vi "Run.vi"(4 "Dispense?":bool, 6 "Pickup_Test_Number":dbl, 7 "Database Entry in":refnum<class "Database Entry.lvclass">, 8 "error in (no error)":errorcluster, 9 "Assembly Type":string, 10 "Control In":T1={"I-O.lvclass"=refnum, "Gantry"=refnum, "Dispenser"="COM1"}, 11 "Assembly In":refnum<class "Assembly Run.lvclass">) -> (0 "error out":errorcluster, 2 "Control Out":T1={"I-O.lvclass"=refnum, "Gantry"=refnum, "Dispenser"="COM1"}, 3 "Assembly Out":refnum<class "Assembly Run.lvclass">, 5 "Database Entry out":refnum<class "Database Entry.lvclass">)   [LabVIEW 2021, in "Assembly Run.lvclass"]
uses:
  Assembly Run.lvclass
  Controller/Controllers.ctl
  Controller/I-O/I-O.lvclass
  C:/Program Files (x86)/Aerotech/A3200/LabVIEW/2010/Bin/Aerotech.A3200.dll
  Program Files (x86)/Aerotech/A3200/LabVIEW/2010/Bin/Aerotech.A3200.dll
  Database Entry/Database Entry.lvclass
  Assembly Run.lvclass/Assembly Run.ctl
  Workspace/Fixture.lvclass
  Routine/Routine.lvclass
  Controller/Motion/Motion.lvclass
  Controller/Motion/A3200/A3200.lvclass
  Drivers/Aerotech A3200/Aerotech.lvlib
  Controller/Controller.lvclass
panel:
  out "Program End?":bool
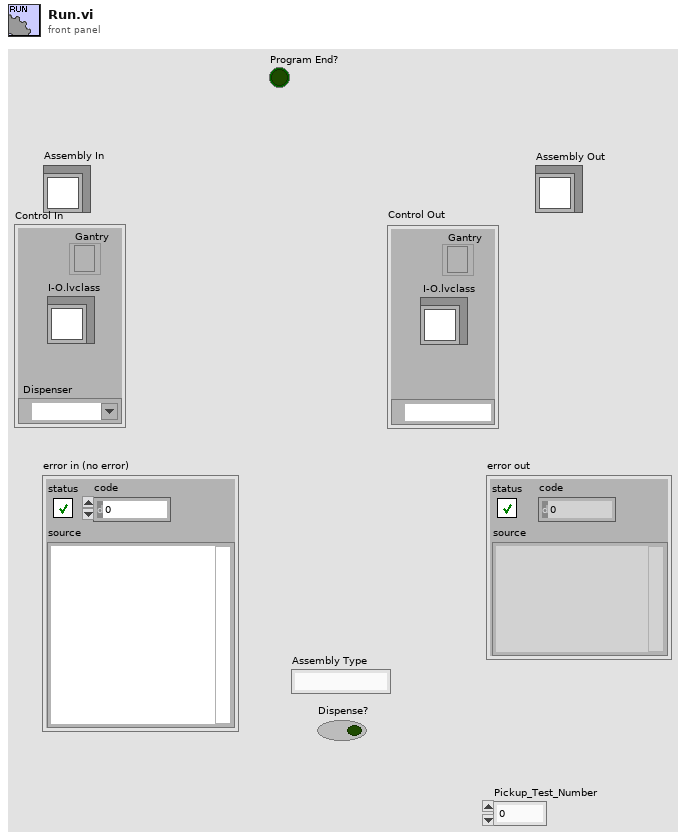
[diagram p1: front panel]
types:
  T1 = typedef "Controller.lvclass/Controllers.ctl" = cluster{"I-O.lvclass":refnum<class "I-O.lvclass">, "Gantry":refnum<k24>, "Dispenser":refnum<visa-resource-name>}
  T2 = typedef "Fixture.lvclass/Workspace.ctl" = cluster{"XYZTheta":dbl[], "Workspace Valve":i32, "Workspace Sensor":i32, "Tray Number":i32, "Position":i32, "Assembly Type":string, "Numeric":dbl, "First Pos":i32}
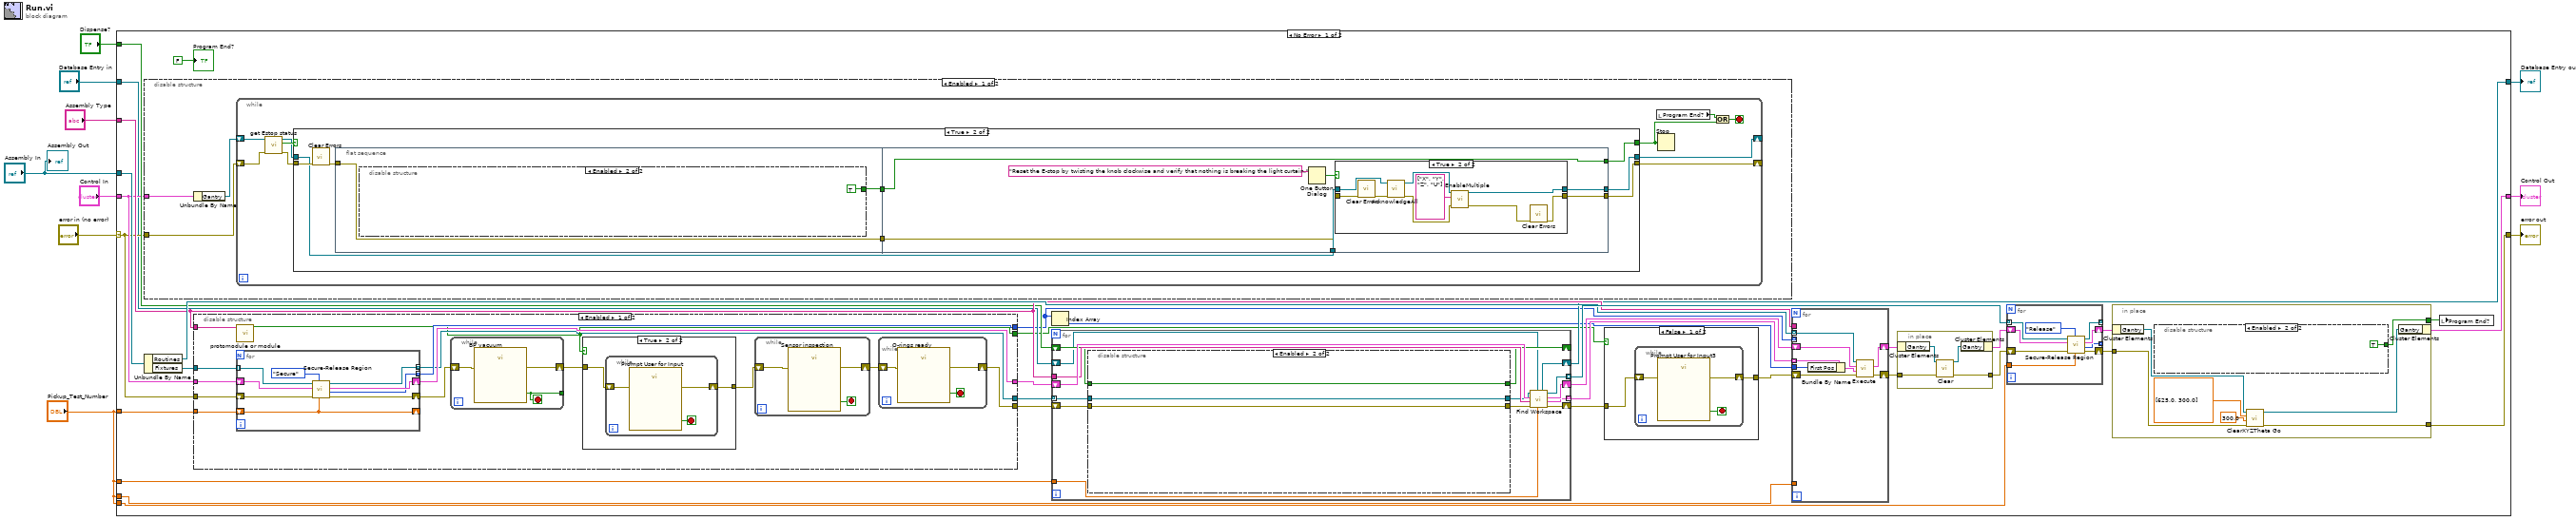
[diagram p0: block diagram]
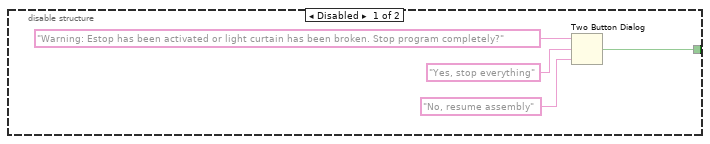
[diagram p4: hidden frame]
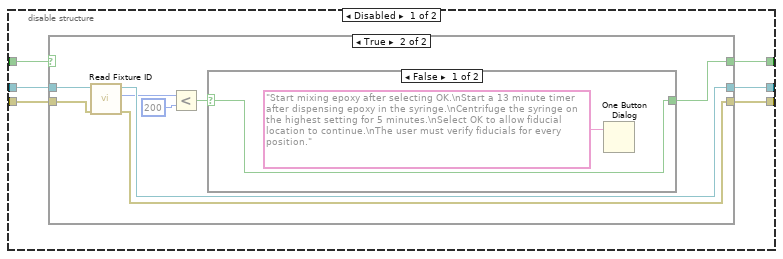
[diagram p7: hidden frame]
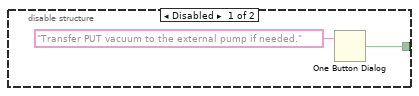
[diagram p10: hidden frame]
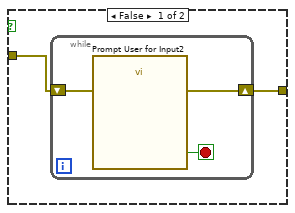
[diagram p11: hidden frame]
diagram:
  n1 = case shown="No Error" "error in (no error)" {
    selector: "error in (no error)" -> [w20 w215]
    tunnel: [w25 w215] -> w9
    tunnel: [w30 w214] -> w8
    tunnel: "Assembly In" -> [w40 _]
    tunnel: "Control In" -> [w21 w214]
    tunnel: "Assembly Type" -> [w23 _]
    tunnel: "Pickup_Test_Number" -> [w36 _]
    tunnel: "Pickup_Test_Number" -> [w34 _]
    tunnel: "Pickup_Test_Number" -> [w35 _]
    tunnel: "Pickup_Test_Number" -> [w33 _]
    tunnel: "Dispense?" -> [w22 _]
    tunnel: "Database Entry in" -> [w17 w213]
    tunnel: [w16 w213] -> w1
    frame No Error {
      n2 = disable-structure shown="Enabled" {
        disable-tunnel: w21 -> [w53 _]
        disable-tunnel: w20 -> [w51 _]
        frame Enabled {
          n3 = Unbundle By Name(w53) -> ("Gantry"=w52:refnum<k24>)
          n4 = while {
            shift-right: [w57] -> _
            shift-left: w52 -> [w63]
            shift-right: [w59] -> _
            shift-left: w51 -> [w62]
            stop <- w56 stop-if-true
            n5 = call "get Estop status.vi"("error in (no error)"=w62, "controller in"=w63) -> ("error out"=w60:errorcluster, "Estop?"=w61:bool, "controller out"=w58:refnum<k24>)  [unwired: 7 in]
            n6 = case shown="True" w61 {
              selector: w61 -> [w65 _]
              tunnel: w60 -> [w66 w74]
              tunnel: [w66 w67] -> w59
              tunnel: [w65 w73] -> w55
              tunnel: w58 -> [w64 w69]
              tunnel: [w64 w68] -> w57
              frame False {
              }
              frame True {
                n7 = call <vilib>:"Clear Errors.vi"("error in (no error)"=w74) -> ("error out"=w71:errorcluster)  [unwired: 5 in, 1 out]
                n8 = flat-sequence {
                  tunnel: [w76] -> w72
                  tunnel: w71 -> [w75]
                  tunnel: [w75] -> w70
                  tunnel: [w88] -> w73
                  tunnel: w72 -> [w88]
                  tunnel: w70 -> [w82]
                  tunnel: w69 -> [w85]
                  tunnel: [w84] -> w68
                  tunnel: [w83] -> w67
                  frame #0 {
                    n9 = disable-structure shown="Enabled" {
                      disable-tunnel: [w77 TRUE ("T button?")] -> w76
                      frame Disabled {
                        n10 = Two Button Dialog(message="Warning: Estop has been activated or light curtain has been broken. Stop program completely?", 1:"No, resume assembly" ("F button name (\"Cancel\")"), 2:"Yes, stop everything" ("T button name (\"OK\")")) -> (T button?=w77:bool)
                      }
                      frame Enabled {
                      }
                    }
                  }
                  frame #1 {
                    n11 = One Button Dialog(message="Reset the E-stop by twisting the knob clockwise and verify that nothing is breaking the light curtain.") -> (true=w86:bool)  [unwired: 1 in]
                    n12 = case shown="True" w86 {
                      tunnel: w85 -> [w90 w98]
                      tunnel: w82 -> [w89 w97]
                      tunnel: [w90 w94] -> w84
                      tunnel: [w89 w91] -> w83
                      frame False {
                      }
                      frame True {
                        n13 = call <vilib>:"Clear Errors.vi"("error in (no error)"=w97) -> ("error out"=w99:errorcluster)  [unwired: 5 in, 1 out]
                        n14 = call "AcknowledgeAll.vi"("error in (no error)"=w99, "controller in"=w98) -> ("error out"=w95:errorcluster, "controller out"=w96:refnum<k24>)  [unwired: 8 in]
                        n15 = call "EnableMultiple.vi"("error in (no error)"=w95, "axis names"=string[] ["X", "Y", "Z", "U"], "controller in"=w96) -> ("error out"=w92:errorcluster, "controller out"=w94:refnum<k24>)  [unwired: 7 in]
                        n16 = call <vilib>:"Clear Errors.vi"("error in (no error)"=w92) -> ("error out"=w91:errorcluster)  [unwired: 5 in, 1 out]
                      }
                    }
                  }
                }
              }
            }
            n17 = local read "Program End?"() -> (w54:bool)
            n18 = Stop(stop? (T)=w55) -> ()
            n19 = Or(x=w54, y=w55) -> (x .or. y?=w56:bool)
          }
        }
        frame Disabled {
        }
      }
      n20 = Unbundle By Name(w40) -> ("Routines"=w24:refnum<class "Routine.lvclass">[], "Fixtures"=w41:refnum<class "Fixture.lvclass">[])
      n21 = disable-structure shown="Enabled" {
        disable-tunnel: [w152 w191] -> w43
        disable-tunnel: w41 -> [w161 w191]
        disable-tunnel: w21 -> [w160 w190]
        disable-tunnel: [w159 w190] -> w37
        disable-tunnel: [w158 _] -> w12
        disable-tunnel: w34 -> [w157 _]
        disable-tunnel: w20 -> [w156 _]
        disable-tunnel: [w149 _] -> w29
        disable-tunnel: w23 -> [w151 _]
        disable-tunnel: [w148 _] -> w13
        frame Enabled {
          n22 = for {
            tunnel: [w189] -> w152 mode=indexing
            tunnel: w161 -> [w188] mode=indexing
            shift-right: [w186] -> w159
            shift-left: w160 -> [w187]
            tunnel: [w184] -> w158 mode=indexing
            shift-right: [w183] -> _
            shift-left: w157 -> [w183]
            shift-right: [w182] -> w155
            shift-left: w156 -> [w181]
            n23 = call-dynamic "Secure-Release Region.vi"("Test Run Number"=w183, "Action"=enum16{"Secure", "Release"}."Secure", "error in (no error)"=w181, "Control In"=w187, "Fixture in"=w188) -> ("error out"=w182:errorcluster, "Position"=w184:i32, "Control Out"=w186:T1, "Fixture out"=w189:refnum<class "Fixture.lvclass">)  [unwired: 3 in]
          }
          n24 = call "protomodule or module.vi"("assembly type"=w151) -> ("protomodule? (T)"=w148:bool)  [unwired: 10 in]
          n25 = while {
            tunnel: [w180] -> _
            shift-right: [w178] -> w154
            shift-left: w155 -> [w179]
            stop <- w180 stop-if-true
            n26 = call "BP vacuum"("error in (no error)"=w179) -> ("BP vacuum is on?"=w180:bool, "error out"=w178:errorcluster)  [unwired: 16 in, 1 out]
          }
          n27 = case shown="True" w148 {
            tunnel: w154 -> [w169 w174]
            tunnel: [w168 w173] -> w153
            frame False {
              n28 = while {
                shift-right: [w171] -> w168
                shift-left: w169 -> [w172]
                stop <- w170 stop-if-true
                n29 = call "Prompt User for Input2"("error in (no error)"=w172) -> ("HB backlighting on?"=w170:bool, "error out"=w171:errorcluster)  [unwired: 16 in, 1 out]
              }
            }
            frame True {
              n30 = while {
                shift-right: [w175] -> w173
                shift-left: w174 -> [w176]
                stop <- w177 stop-if-true
                n31 = call "Prompt User for Input"("error in (no error)"=w176) -> ("BP paper is removed?"=w177:bool, "error out"=w175:errorcluster)  [unwired: 16 in, 1 out]
              }
            }
          }
          n32 = while {
            shift-right: [w163] -> w150
            shift-left: w153 -> [w162]
            stop <- w164 stop-if-true
            n33 = call "Sensor inspection"("error in (no error)"=w162) -> ("Sensors inspected?"=w164:bool, "error out"=w163:errorcluster)  [unwired: 16 in, 1 out]
          }
          n34 = while {
            shift-right: [w166] -> w149
            shift-left: w150 -> [w165]
            stop <- w167 stop-if-true
            n35 = call "O-rings ready"("error in (no error)"=w165) -> ("O-rings ready?"=w167:bool, "error out"=w166:errorcluster)  [unwired: 16 in, 1 out]
          }
        }
        frame Disabled {
        }
      }
      n36 = Index Array(array=w12) -> (element=w11:i32)  [unwired: 1 in]
      n37 = for {
        tunnel: w43 -> [w107] mode=indexing
        tunnel: [w110] -> w44 mode=indexing
        tunnel: [w114] -> w32 mode=indexing
        shift-right: [w112] -> w39
        shift-left: w37 -> [w113]
        tunnel: w23 -> [w111]
        tunnel: w33 -> [w109]
        shift-right: [w108] -> w15
        shift-left: w29 -> [w105]
        shift-right: [w102] -> _
        shift-left: w22 -> [w103]
        shift-right: [w100] -> w16
        shift-left: w17 -> [w101]
        n38 = disable-structure shown="Enabled" {
          disable-tunnel: w107 -> [w120 w137]
          disable-tunnel: [w119 w137] -> w106
          disable-tunnel: w105 -> [w118 w136]
          disable-tunnel: [w117 w136] -> w104
          disable-tunnel: w103 -> [w116 w135]
          disable-tunnel: [w115 w135] -> w102
          frame Disabled {
            n39 = case shown="True" w116 {
              selector: w116 -> [w121 _]
              tunnel: w120 -> [w123 w131]
              tunnel: [w123 w130] -> w119
              tunnel: w118 -> [w122 w129]
              tunnel: [w122 w128] -> w117
              tunnel: [w121 w124] -> w115
              frame False {
              }
              frame True {
                n40 = call "Read Fixture ID.vi"("error in (no error)"=w129, "Fixture in"=w131) -> ("error out"=w128:errorcluster, "Fixture ID"=w127:i32, "Fixture out"=w130:refnum<class "Fixture.lvclass">)  [unwired: 7 in]
                n41 = Less?(x=w127, y=200) -> (x < y?=w125:bool)
                n42 = case shown="False" w125 {
                  selector: w125 -> [w132 w134]
                  tunnel: [w132 w134] -> w124
                  frame False {
                    n43 = One Button Dialog(message="Start mixing epoxy after selecting OK.\nStart a 13 minute timer after dispensing epoxy in the syringe.\nCentrifuge the syringe on the highest setting for 5 minutes.\nSelect OK to allow fiducial location to continue.\nThe user must verify fiducials for every position.") -> ()  [unwired: 1 in, 1 out]
                  }
                  frame True {
                  }
                }
              }
            }
          }
          frame Enabled {
          }
        }
        n44 = call-dynamic "Find Workspace.vi"("Pickup_Test_Number"=w109, "Database Entry in"=w101, "Error In"=w104, "Assembly Type"=w111, "Control In"=w113, "Workspace In"=w106) -> ("Error Out"=w108:errorcluster, 1:"Workspace Out"=w110:T2, "Control Out"=w112:T1, 3:"Workspace Out"=w114:refnum<class "Fixture.lvclass">, "Database Entry out"=w100:refnum<class "Database Entry.lvclass">)  [unwired: 1 in]
      }
      n45 = case shown="False" w13 {
        tunnel: w15 -> [w46 w50]
        tunnel: [w45 w50] -> w14
        frame False {
          n46 = while {
            shift-right: [w48] -> w45
            shift-left: w46 -> [w49]
            stop <- w47 stop-if-true
            n47 = call "Prompt User for Input3"("error in (no error)"=w49) -> ("HB backlighting off?"=w47:bool, "error out"=w48:errorcluster)  [unwired: 16 in, 1 out]
          }
        }
        frame True {
        }
      }
      n48 = for {
        tunnel: w24 -> [w212] mode=indexing
        tunnel: w44 -> [w207] mode=indexing
        shift-right: [w210] -> w38
        shift-left: w39 -> [w211]
        tunnel: w23 -> [_]
        tunnel: w12 -> [_] mode=indexing
        tunnel: w35 -> [_]
        shift-right: [w208] -> w28
        shift-left: w14 -> [w209]
        tunnel: w11 -> [w205]
        n49 = Bundle By Name(cluster=w207, "First Pos"=w205) -> (w206:T2)
        n50 = call-dynamic "Execute.vi"("error in (no error)"=w209, "Workspace"=w206, "Control In"=w211, "Routine in"=w212) -> ("error out"=w208:errorcluster, "Control Out"=w210:T1)  [unwired: 5 in, 1 out]
      }
      n51 = in-place {
        in-place-border: w28 -> [w202]
        in-place-border: [w201] -> w27
        n52 = in-place-cluster #1(w38) -> ("Gantry"=w203:refnum<k24>)
        n53 = call "Clear.vi"("error in (no error)"=w202, "Gantry In"=w203) -> ("error out"=w201:errorcluster, "Gantry Out"=w204:refnum<k24>)  [unwired: 8 in]
        n54 = in-place-cluster #1("Gantry"=w204) -> (w42:T1)
      }
      n55 = for {
        tunnel: w32 -> [w200] mode=indexing
        shift-right: [w199] -> w31
        shift-left: w42 -> [w198]
        tunnel: w36 -> [w196]
        tunnel: [w195] -> _ mode=indexing
        tunnel: [w194] -> _ mode=indexing
        shift-right: [w192] -> w26
        shift-left: w27 -> [w193]
        n56 = call-dynamic "Secure-Release Region.vi"("Test Run Number"=w196, "Action"=enum16{"Secure", "Release"}."Release", "error in (no error)"=w193, "Control In"=w198, "Fixture in"=w200) -> ("error out"=w192:errorcluster, "Position"=w195:i32, "Control Out"=w199:T1, "Fixture out"=w194:refnum<class "Fixture.lvclass">)  [unwired: 3 in]
      }
      n57 = in-place {
        in-place-border: w26 -> [w140]
        in-place-border: [w139] -> w25
        in-place-border: [w138] -> w18
        n58 = in-place-cluster #2(w31) -> ("Gantry"=w143:refnum<k24>)
        n59 = disable-structure shown="Enabled" {
          disable-tunnel: [w145 TRUE ("true")] -> w138
          frame Disabled {
            n60 = One Button Dialog(message="Transfer PUT vacuum to the external pump if needed.") -> (true=w145:bool)  [unwired: 1 in]
          }
          frame Enabled {
          }
        }
        n61 = call "ClearXYZTheta Go.vi"("error in (no error)"=w140, "Speed"=300.0, "XYZTheta In"=dbl[] [625.0, 300.0], "Gantry In"=w143) -> ("error out"=w139:errorcluster, "Gantry Out"=w142:refnum<k24>)  [unwired: 5 in, 1 out]
        n62 = in-place-cluster #2("Gantry"=w142) -> (w30:T1)
      }
      n63 = local write "Program End?"(w18) -> ()
      "Program End?" <- FALSE ("Program End?")
    }
    frame Error {
    }
  }
  "error out" <- w9
  "Control Out" <- w8
  "Database Entry out" <- w1
  "Assembly Out" <- "Assembly In"
